vi "Read DataSocket Mode.vi"(8 "error in (no error)":errorcluster, 11 "Control.lvclass in":refnum<class "Control.lvclass">) -> (0 "error out":errorcluster, 2 "DtSktMode":T1(ring), 3 "Control.lvclass out":refnum<class "Control.lvclass">)   [LabVIEW 2015, in "Control.lvclass"]
uses:
  Control.lvclass
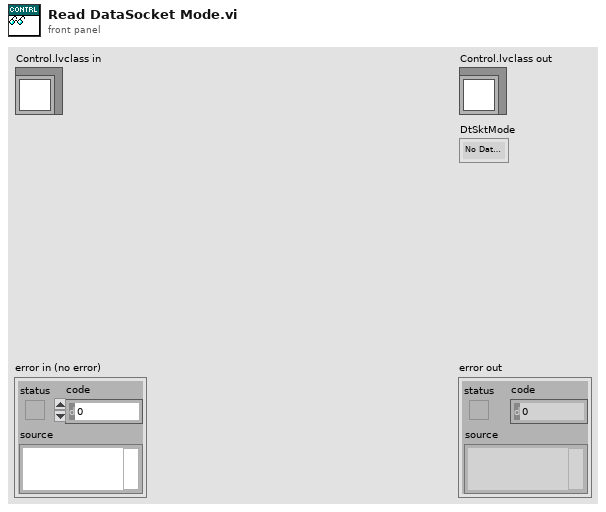
[diagram p1: front panel]
types:
  T1 = enum32{"No DataSocket", "Publish", "Subscribe", "Publish & Subscribe"}
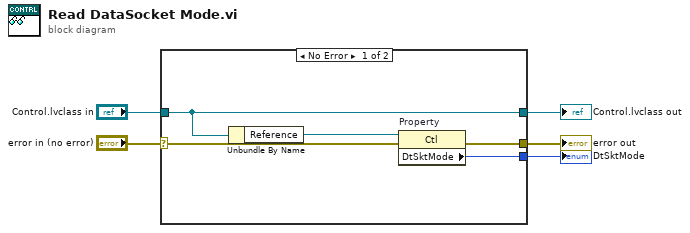
[diagram p0: block diagram]
diagram:
  n1 = case shown="No Error" "error in (no error)" {
    selector: "error in (no error)" -> [w6 w12]
    tunnel: [w9 w12] -> w4
    tunnel: [w8 w11] -> w2
    tunnel: "Control.lvclass in" -> [w8 w11]
    tunnel: [w10 _] -> w1
    frame No Error {
      n2 = Unbundle By Name(w8) -> ("Reference"=w7:refnum<vi>)
      n3 = property on="Property" class="Ctl"(reference=w7, error in=w6) -> (error out=w9:errorcluster, "DtSktMode"=w10:T1)  [unwired: 1 out]
    }
    frame Error {
    }
  }
  "error out" <- w4
  "Control.lvclass out" <- w2
  "DtSktMode" <- w1
